vi "Image Tester.vi"(11 "Particle Report":T1) -> (3 "Positive":bool)   [LabVIEW 2017]
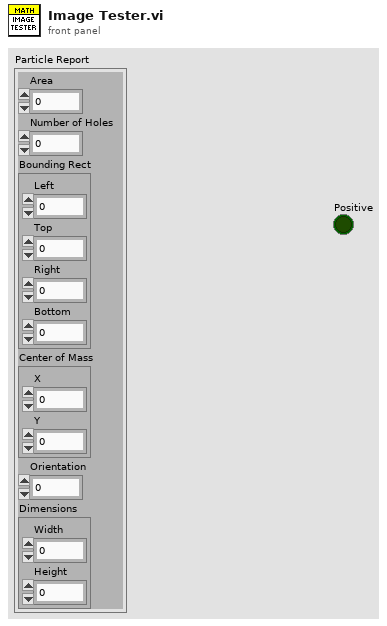
[diagram p1: front panel]
types:
  T1 = cluster{"Area":dbl, "Number of Holes":dbl, "Bounding Rect":cluster{"Left":dbl, "Top":dbl, "Right":dbl, "Bottom":dbl}, "Center of Mass":cluster{"X":dbl, "Y":dbl}, "Orientation":dbl, "Dimensions":cluster{"Width":dbl, "Height":dbl}}
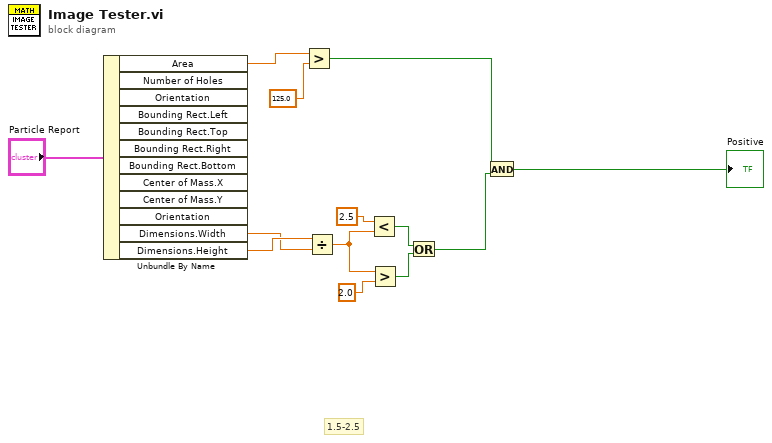
[diagram p0: block diagram]
diagram:
  # "1.5-2.5"
  n1 = Unbundle By Name("Particle Report") -> ("Area"=w1:dbl, "Dimensions.Width"=w11:dbl, "Dimensions.Height"=w12:dbl)  [unwired: 9 out]
  n2 = Greater?(x=w1, y=125.0 ("x")) -> (0:w5:bool)
  n3 = Divide(x=w12, y=w11) -> (x/y=w8:dbl)
  n4 = Less?(x=2.5, y=w8) -> (x < y?=w10:bool)
  n5 = Greater?(x=w8, y=2.0) -> (0:w9:bool)
  n6 = Or(x=w10, y=w9) -> (x .or. y?=w4:bool)
  n7 = And(x=w5, y=w4) -> (x .and. y?=→"Positive":bool)
